vi "ADAM 5000 Relay Control.vi"(9 "State":bool=TRUE, 10 "Relay # (1=1st relay)":i32, 11 "Remote IP Address 2":string="192.168.11.50") -> ()   [LabVIEW 2016]
uses:
  nimodbus121/71/vi.lib/NI Modbus.llb/MB Modbus Command.ctl
panel:
  in  "Modbus Command":T1={"Function Code"=15, "Starting Address"=17, "Quantity"=1, "Data"=[], "Discrete"=[]} {"Function Code" items=["Read Coils"=1, "Read Discrete Inputs"=2, "Read Holding Registers"=3, "Read Input Registers"=4, "Write Single Coil"=5, "Write Single Register"=6, "Read Exception Status"=7, "Write Multiple Coils"=15, "Write Multiple Registers"=16]}
  in  "Remote Port 2":u16=502
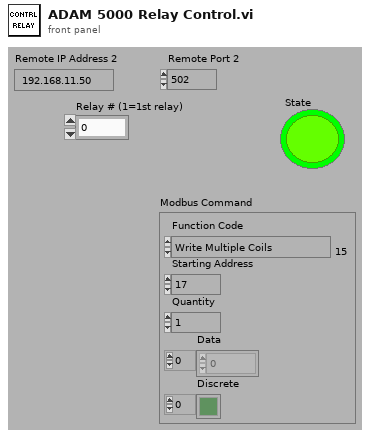
[diagram p1: front panel]
types:
  T1 = typedef "MB Modbus Command.ctl" = cluster{"Function Code":u8, "Starting Address":u16, "Quantity":u16, "Data":u16[], "Discrete":bool[]}
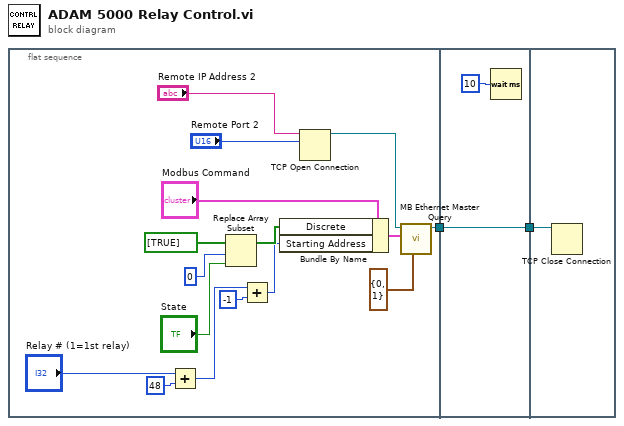
[diagram p0: block diagram]
diagram:
  n1 = flat-sequence {
    tunnel: [w6] -> w2
    tunnel: w2 -> [w20]
    tunnel: [w20] -> w1
    tunnel: w1 -> [w21]
    frame #0 {
      n2 = Add(x="Relay # (1=1st relay)", y=48) -> (x+y=w3:i32)
      n3 = Replace Array Subset(array=bool[] [TRUE] ("Discrete"), new element="State", index=0) -> (w10:bool[])
      n4 = Add(x=w3, y=-1) -> (x+y=w8:i32)
      n5 = Bundle By Name(cluster="Modbus Command", "Discrete"=w10, "Starting Address"=w8) -> (w15:T1)
      n6 = TCP Open Connection(address="Remote IP Address 2", remote port or service name="Remote Port 2") -> (connection ID=w16:refnum<k5>)  [unwired: 3 in, 1 out]
      n7 = call "MB Ethernet Master Query.vi"("MBAP Header"=cluster{"Transaction ID":u16, "Unit ID":u8} {"Transaction ID"=0, "Unit ID"=1}, "Modbus Command"=w15, "TCP Connection Refnum in"=w16) -> ("TCP Connection Refnum (dup)"=w6:refnum<k5>)  [unwired: 4 in, 4 out]
    }
    frame #1 {
      n8 = Wait (ms)(milliseconds to wait=u32 10) -> ()  [unwired: 1 out]
    }
    frame #2 {
      n9 = TCP Close Connection(connection ID=w21) -> ()  [unwired: 2 in, 2 out]
    }
  }
